vi "Grab Scrollback Lines.vi"(8 "error in (no error)":errorcluster, 10 "Count":i32, 11 "TermBuffer in":refnum<class "TermBuffer.lvclass">) -> (0 "error out":errorcluster, 2 "Lines":refnum<class "TermLine.lvclass">[](array[class]), 3 "TermBuffer out":refnum<class "TermBuffer.lvclass">)   [LabVIEW 2020, in "Terminal.lvlib" / "TermBuffer.lvclass"]
uses:
  TermBuffer.lvclass
  TermBuffer.lvclass/TermBuffer.ctl
  TermLine/TermLine.lvclass
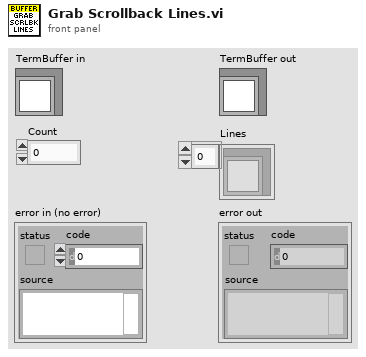
[diagram p1: front panel]
types:
  T1 = typedef "Terminal.lvlib/TermBuffer.lvclass/Ref Data.ctl" = cluster{"Lines":refnum<class "TermLine.lvclass">[]}
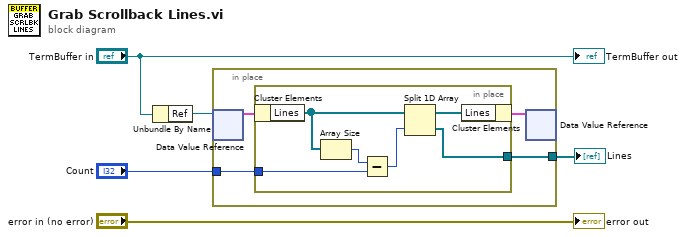
[diagram p0: block diagram]
diagram:
  n1 = Unbundle By Name("TermBuffer in") -> ("Ref"=w4:refnum<data-value>)
  n2 = in-place {
    in-place-border: "Count" -> [w7]
    in-place-border: [w6] -> w1
    n3 = in-place-dvr #1(w4) -> (w9:T1)  [unwired: 1 out]
    n4 = in-place {
      in-place-border: w7 -> [w14]
      in-place-border: [w10] -> w6
      n5 = in-place-cluster #2(w9) -> ("Lines"=w13:refnum<class "TermLine.lvclass">[])
      n6 = Array Size(array=w13) -> (size(s)=w15:i32)
      n7 = Subtract(x=w15, y=w14) -> (x-y=w12:i32)
      n8 = Split 1D Array(array=w13, index=w12) -> (first subarray=w11:refnum<class "TermLine.lvclass">[], second subarray=w10:refnum<class "TermLine.lvclass">[])
      n9 = in-place-cluster #2("Lines"=w11) -> (w8:T1)
    }
    n10 = in-place-dvr #1(w8) -> ()  [unwired: 2 out]
  }
  "Lines" <- w1
  "error out" <- "error in (no error)"
  "TermBuffer out" <- "TermBuffer in"
